vi "Render Stats.vi"(8 "error in (no error)":errorcluster, 11 "Main Controller Actor in":refnum<class "Main Controller Actor.lvclass">) -> (0 "error out":errorcluster, 3 "Renderer out":refnum<class "Renderer.lvclass">)   [LabVIEW 2021, in "Main Controller Actor.lvclass"]
uses:
  Main Controller Actor.lvclass
  Main Controller Actor.lvclass/Main Controller Actor.ctl
  Resource Manager/Resource Manager.lvclass
  Renderer/Renderer.lvclass
  Re-use Libraries/Vector 2D/Vector 2D.lvclass
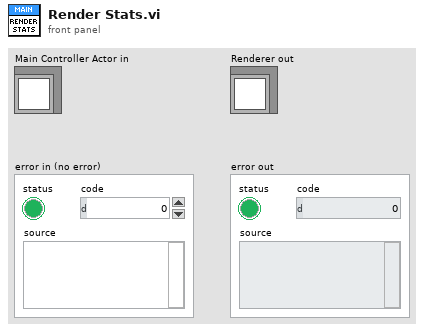
[diagram p1: front panel]
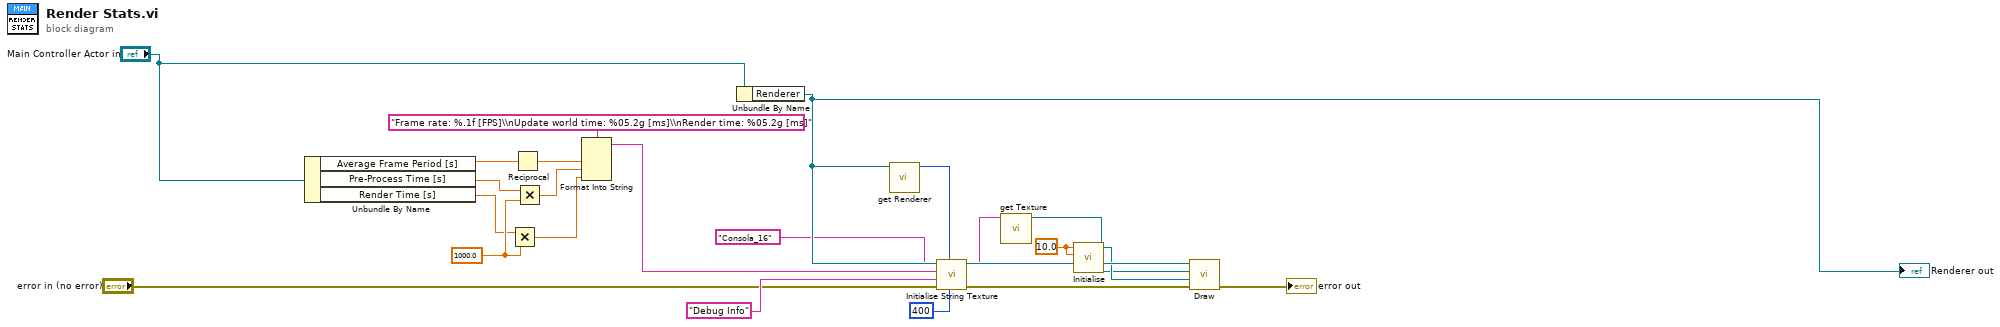
[diagram p0: block diagram]
diagram:
  w16 = sgl 10.0 ("x")
  w12 = 1000.0 ("y")
  n1 = Unbundle By Name("Main Controller Actor in") -> ("Average Frame Period [s]"=w6:dbl, "Pre-Process Time [s]"=w11:dbl, "Render Time [s]"=w7:dbl)
  n2 = Multiply(x=w7, y=w12) -> (x*y=w13:dbl)
  n3 = Reciprocal(x=w6) -> (1/x=w9:dbl)
  n4 = Multiply(x=w11, y=w12) -> (x*y=w14:dbl)
  n5 = Format Into String(format string="Frame rate: %.1f [FPS]\\nUpdate world time: %05.2g [ms]\\nRender time: %05.2g [ms]", w9, w14, w13) -> (resulting string=w8:string)  [unwired: 2 in, 1 out]
  n6 = Unbundle By Name("Main Controller Actor in") -> ("Renderer"=w21:refnum<class "Renderer.lvclass">)
  "Renderer out" <- w21
  n7 = call-dynamic "get Renderer.vi"("Renderer in"=w21) -> ("Renderer"=w22:u32)  [unwired: 10 in]
  n8 = call "Initialise String Texture.vi"("Wrap Length [pixels]"=400, "Renderer"=w22, "error in (no error)"="error in (no error)", "Name"="Debug Info", "Text"=w8, "Font Combo"="Consola_16") -> ("error out"=w19:errorcluster, "Name In Cache"=w3:string)  [unwired: 4 in]
  n9 = call "get Texture.vi"("Texture Name"=w3) -> ("Texture"=w15:refnum<class "Texture.lvclass">)  [unwired: 10 in]
  n10 = call "Initialise.vi"("y"=w16, "x"=w16) -> ("Vector 2D out"=w17:refnum<class "Vector 2D.lvclass">)  [unwired: 9 in]
  n11 = call "Draw.vi"("error in (no error)"=w19, "Destination"=w17, "Texture"=w15, "Renderer"=w21) -> ("error out"=→"error out":errorcluster)  [unwired: 7 in]
